vi "Heure.vi"() -> (3 "chaîne concaténée":string)   [LabVIEW 2020]
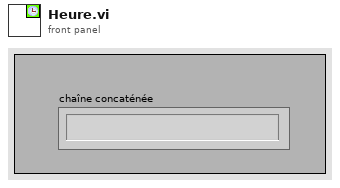
[diagram p1: front panel]
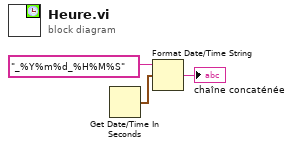
[diagram p0: block diagram]
diagram:
  n1 = Get Date/Time In Seconds() -> (seconds since 1Jan1904=w3:timestamp)
  n2 = Format Date/Time String(time format string (%c)="_%Y%m%d_%H%M%S" ("chaîne de format de l'heure (%c)"), seconds (now)=w3) -> (date/time string=→"chaîne concaténée":string)  [unwired: 1 in]
